vi "Select_Card_tl.vi"(1 "Card number":i32(slide) max=7 step=1 scale=0.0..7.0) -> ()   [LabVIEW 2010]
panel:
  out "?":string
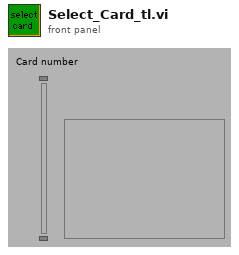
[diagram p1: front panel]
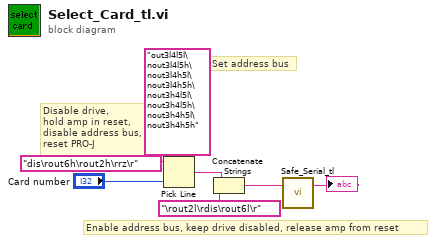
[diagram p0: block diagram]
diagram:
  # "Set address bus"
  # "Enable address bus, keep drive disabled, release amp from reset"
  # "Disable drive,\nhold amp in reset,\ndisable address bus,\nreset PRO-J"
  n1 = Pick Line(string ("")="dis\rout6h\rout2h\rrz\r", multi-line string="out3l4l5l\nout3l4l5h\nout3l4h5l\nout3l4h5h\nout3h4l5l\nout3h4l5h\nout3h4h5l\nout3h4h5h", line index="Card number") -> (output string=w5:string)
  n2 = Concatenate Strings(w5, "\rout2l\rdis\rout6l\r") -> (w1:string)
  n3 = call "Safe_Serial_tl.vi"("Tx String"=w1) -> ("Rx String"=→"?":string)  [unwired: 5 in, 1 out]
